vi "Connect.vi"(8 "error in":errorcluster, 11 "WAMP Client in":refnum<class "WAMP Client.lvclass">) -> (0 "error out":errorcluster, 3 "WAMP Client out":refnum<class "WAMP Client.lvclass">)   [LabVIEW 2020, in "wamplv.lvlib" / "WAMP Client.lvclass"]
doc: "Connects to the WAMP router and performs the HELLO/WELCOME handshake. After calling this the WAMP session is ready for use."
uses:
  WAMP Client.lvclass
  WAMP Client.lvclass/WAMP Client.ctl
  Private/TypeDef/Termination Reason.ctl
  Private/TypeDef/Termination Reason Enum.ctl
  <vilib>/JDP Science/JSONtext/Get Array Elements.vi
  Private/Loops/Daemon.vi
  Private/Comm Handlers/ICommHandler/ICommHandler.lvclass
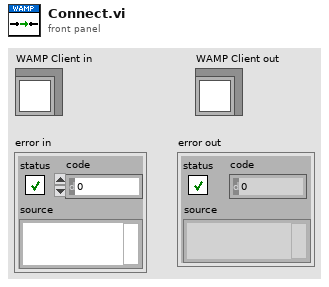
[diagram p1: front panel]
types:
  T1 = typedef "wamplv.lvlib/WAMP Client.lvclass/Termination Reason.ctl" = cluster{"Reason":T2, "Reason URI":string, "Message":string}
  T2 = typedef "wamplv.lvlib/WAMP Client.lvclass/Termination Reason Enum.ctl" = enum16{"Goodbye Received", "Abort Received", "Send Goodbye", "Send Abort", "Read Loop Failure", "Write Loop Failure", "Message Loop Failure"}
  T3 = typedef "wamplv.lvlib/WAMP Client.lvclass/WAMP Received Message.ctl" = cluster{"Message JSON":string[], "Message Codes":T4}
  T4 = typedef "wamplv.lvlib/WAMP Client.lvclass/WAMP Message Codes.ctl" = u16
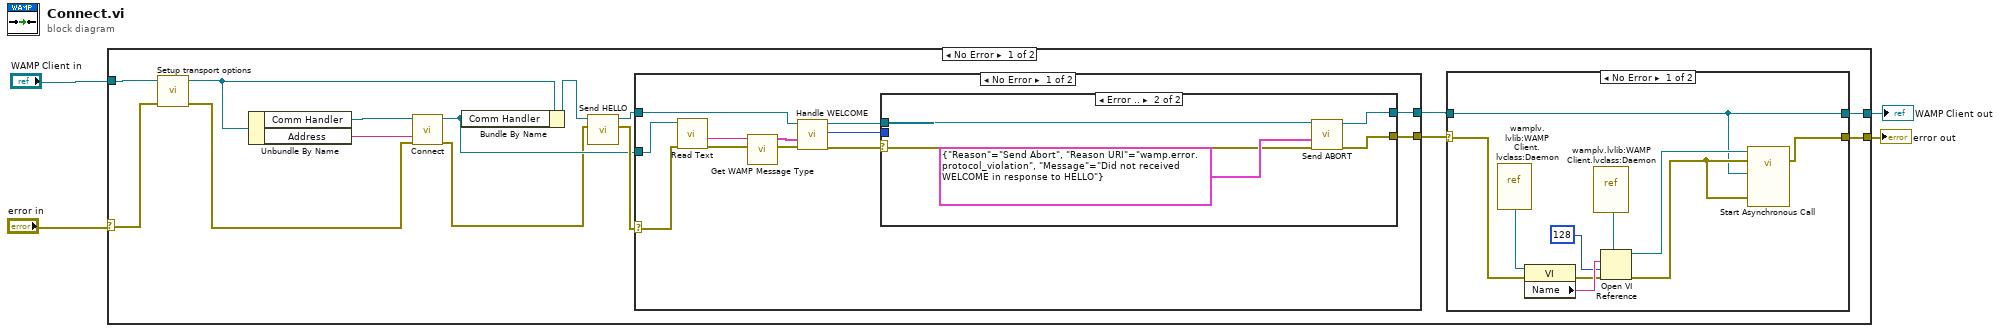
[diagram p0: block diagram]
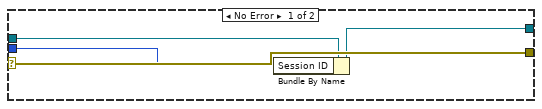
[diagram p3: hidden frame]
diagram:
  n1 = case shown="No Error" "error in" {
    selector: "error in" -> [w6 w56]
    tunnel: [w13 w56] -> w3
    tunnel: [w11 w55] -> w1
    tunnel: "WAMP Client in" -> [w7 w55]
    frame No Error {
      n2 = call "Setup transport options.vi"("error in (no error)"=w6, "WAMP Client in"=w7) -> ("error out"=w5:errorcluster, "WAMP Client out"=w8:refnum<class "WAMP Client.lvclass">)  [unwired: 8 in]
      n3 = Unbundle By Name(w8) -> ("Comm Handler"=w17:refnum<class "ICommHandler.lvclass">, "Address"=w16:string)
      n4 = call-dynamic "Connect.vi"("error in"=w5, "Address"=w16, "ICommHandler in"=w17) -> ("error out"=w12:errorcluster, "ICommHandler out"=w14:refnum<class "ICommHandler.lvclass">)  [unwired: 5 in]
      n5 = Bundle By Name(cluster=w8, "Comm Handler"=w14) -> (w15:refnum<class "WAMP Client.lvclass">)
      n6 = call-dynamic "Send HELLO.vi"("error in (no error)"=w12, "WAMP Client in"=w15) -> ("error out"=w19:errorcluster, "WAMP Client out"=w18:refnum<class "WAMP Client.lvclass">)  [unwired: 8 in]
      n7 = case shown="No Error" w19 {
        selector: w19 -> [w35 w53]
        tunnel: w18 -> [w41 w54]
        tunnel: [w38 w54] -> w10
        tunnel: [w40 w53] -> w9
        tunnel: w14 -> [w43 _]
        frame No Error {
          n8 = call-dynamic "Read Text.vi"("error in (no error)"=w35, "ICommHandler in"=w43) -> ("error out"=w34:errorcluster, "String"=w42:string)  [unwired: 5 in, 1 out]
          n9 = call "Get WAMP Message Type.vi"("error in (no error)"=w34, "JSON"=w42) -> ("error out"=w32:errorcluster, "WAMP Message"=w36:T3)  [unwired: 6 in, 2 out]
          n10 = call-dynamic "Handle WELCOME.vi"("error in (no error)"=w32, "WAMP Message"=w36, "WAMP Client in"=w41) -> ("error out"=w33:errorcluster, "Session ID"=w37:u64, "WAMP Client out"=w39:refnum<class "WAMP Client.lvclass">)  [unwired: 6 in]
          n11 = case shown="Error .." w33 {
            selector: w33 -> [w47 w49]
            tunnel: [w47 w48] -> w40
            tunnel: w39 -> [w44 w52]
            tunnel: [w46 w51] -> w38
            tunnel: w37 -> [w45 _]
            frame No Error {
              n12 = Bundle By Name(cluster=w44, "Session ID"=w45) -> (w46:refnum<class "WAMP Client.lvclass">)
            }
            frame Error {
              n13 = call-dynamic "Send ABORT.vi"("error in (no error)"=w49, "Abort Request"=T1 {"Reason"=enum."Send Abort", "Reason URI"="wamp.error.protocol_violation", "Message"="Did not received WELCOME in response to HELLO"} ("Termination Reason"), "WAMP Client in"=w52) -> ("error out"=w48:errorcluster, "WAMP Client out"=w51:refnum<class "WAMP Client.lvclass">)  [unwired: 7 in]
            }
          }
        }
        frame Error {
        }
      }
      n14 = case shown="No Error" w9 {
        selector: w9 -> [w22 w30]
        tunnel: [w25 w30] -> w13
        tunnel: w10 -> [w20 w31]
        tunnel: [w20 w31] -> w11
        frame No Error {
          n15 = vi-ref "wamplv.lvlib:WAMP Client.lvclass:Daemon.vi"() -> (w28:refnum<vi>)
          n16 = property class="VI"(reference=w28, error in=w22) -> (error out=w23:errorcluster, "Name"=w26:string)  [unwired: 1 out]
          n17 = vi-ref "wamplv.lvlib:WAMP Client.lvclass:Daemon.vi"() -> (w27:refnum<vi>)
          n18 = Open VI Reference(type specifier VI Refnum (for type only)=w27, vi path=w26, options=128, error in (no error)=w23) -> (vi reference=w29:refnum<vi>, error out=w21:errorcluster)  [unwired: 2 in]
          n19 = call-by-ref "Start Asynchronous Call"(reference=w29, error in=w21, 8:"error in (no error)"=w21, "WAMP Client in"=w20) -> (error out=w25:errorcluster)  [unwired: 8 in, 3 out]
        }
        frame Error {
        }
      }
    }
    frame Error {
    }
  }
  "error out" <- w3
  "WAMP Client out" <- w1
